vi "DY_VI_ref.vi"(1 "EQUIP LIST":string[](array[string])) -> (0 "VI_ref":refnum<vi>[](array[refnum]))   [LabVIEW 2024, in "Launcher_DTU.lvlib"]
uses:
  Launcher_DTU.lvlib
  Modules/Barcode_Scanner/Barcode Scanner.vi
  Modules/Keyence/Keyence_VS150.vi
  Modules/Power_Supply/MP711134-14V.vi
  Modules/Power_Supply-2/Multicom_MP711134-12V/MP711134-12V.vi
  Modules/Keysight_34461a/Keysight34461a.vi
  Modules/DMM6500/DMM6500.vi
  Modules/PCANusb_DTU/PCAN.vi
  Modules/ADAM_DI/ADAM_DI.vi
  Modules/Relay_Module/Relay_Module.vi
  Modules/Neoway_flashing/Noeway_Flashing.vi
  Modules/MCU_Flashing/MCU_Flashing.vi
  Modules/Barcode_Scanner/Barcode_Scanner.lvlib
  Modules/Keyence/Keyence_VS150.lvlib
  Modules/Keysight_34461a/Keysight_34461a.lvlib
  Modules/PCANusb_DTU/PCANusb_DTU.lvlib
  Modules/DMM6500/DMM6500.lvlib
  Modules/Power_Supply-2/Multicom_MP711134-12V/Multicom_MP711134-12V.lvlib
  Modules/Power_Supply/Multicom_MP711134-14V.lvlib
  Modules/ADAM_DI/ADAM_DI.lvlib
  Modules/Relay_Module/Relay_Module.lvlib
  Modules/Neoway_flashing/Neoway_flashing.lvlib
  Modules/MCU_Flashing/MCU_Flashing.lvlib
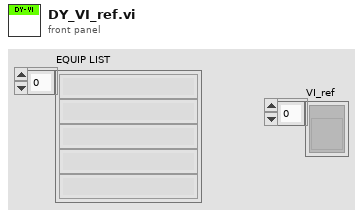
[diagram p1: front panel]
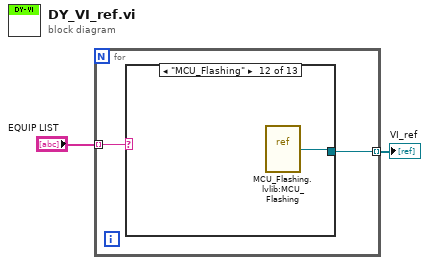
[diagram p0: block diagram]
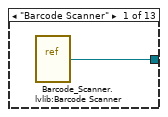
[diagram p2: hidden frame]
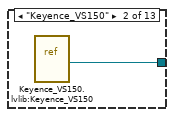
[diagram p3: hidden frame]
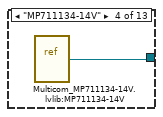
[diagram p5: hidden frame]
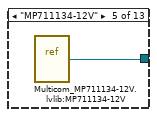
[diagram p6: hidden frame]
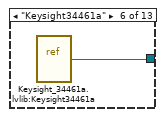
[diagram p7: hidden frame]
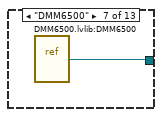
[diagram p8: hidden frame]
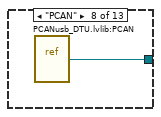
[diagram p9: hidden frame]
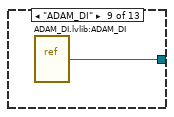
[diagram p10: hidden frame]
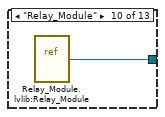
[diagram p11: hidden frame]
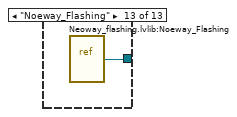
[diagram p13: hidden frame]
diagram:
  n1 = for {
    tunnel: "EQUIP LIST" -> [w4] mode=indexing
    tunnel: [w3] -> w1 mode=indexing
    n2 = case shown="\"MCU_Flashing\"" w4 {
      tunnel: [w5 w6 _ w7 w8 w9 w10 w11 w12 w13 _ w14 w15] -> w3
      frame "Barcode Scanner" {
        n3 = vi-ref "Barcode_Scanner.lvlib:Barcode Scanner.vi"() -> (w5:refnum<vi>)
      }
      frame "Keyence_VS150" {
        n4 = vi-ref "Keyence_VS150.lvlib:Keyence_VS150.vi"() -> (w6:refnum<vi>)
      }
      frame "Printer" {
      }
      frame "MP711134-14V" {
        n5 = vi-ref "Multicom_MP711134-14V.lvlib:MP711134-14V.vi"() -> (w7:refnum<vi>)
      }
      frame "MP711134-12V" {
        n6 = vi-ref "Multicom_MP711134-12V.lvlib:MP711134-12V.vi"() -> (w8:refnum<vi>)
      }
      frame "Keysight34461a" {
        n7 = vi-ref "Keysight_34461a.lvlib:Keysight34461a.vi"() -> (w9:refnum<vi>)
      }
      frame "DMM6500" {
        n8 = vi-ref "DMM6500.lvlib:DMM6500.vi"() -> (w10:refnum<vi>)
      }
      frame "PCAN" {
        n9 = vi-ref "PCANusb_DTU.lvlib:PCAN.vi"() -> (w11:refnum<vi>)
      }
      frame "ADAM_DI" {
        n10 = vi-ref "ADAM_DI.lvlib:ADAM_DI.vi"() -> (w12:refnum<vi>)
      }
      frame "Relay_Module" {
        n11 = vi-ref "Relay_Module.lvlib:Relay_Module.vi"() -> (w13:refnum<vi>)
      }
      frame Default {
      }
      frame "MCU_Flashing" {
        n12 = vi-ref "MCU_Flashing.lvlib:MCU_Flashing.vi"() -> (w14:refnum<vi>)
      }
      frame "Noeway_Flashing" {
        n13 = vi-ref "Neoway_flashing.lvlib:Noeway_Flashing.vi"() -> (w15:refnum<vi>)
      }
    }
  }
  "VI_ref" <- w1
